vi "ParseCharacters.vi"(11 "TextIn":string) -> (3 "Characters":T1[](array[typedef]))   [LabVIEW 2022 SP3]
uses:
  <vilib>/Utility/error.llb/Trim Whitespace One-Sided.vi
  TypeDefs/Character.ctl
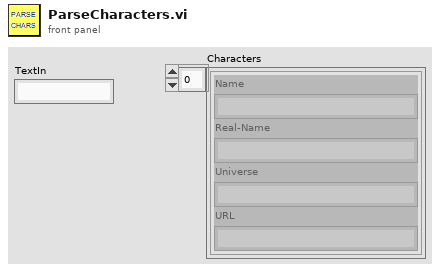
[diagram p1: front panel]
types:
  T1 = typedef "Character.ctl" = cluster{"Name":string, "Real-Name":string, "Universe":string, "URL":string}
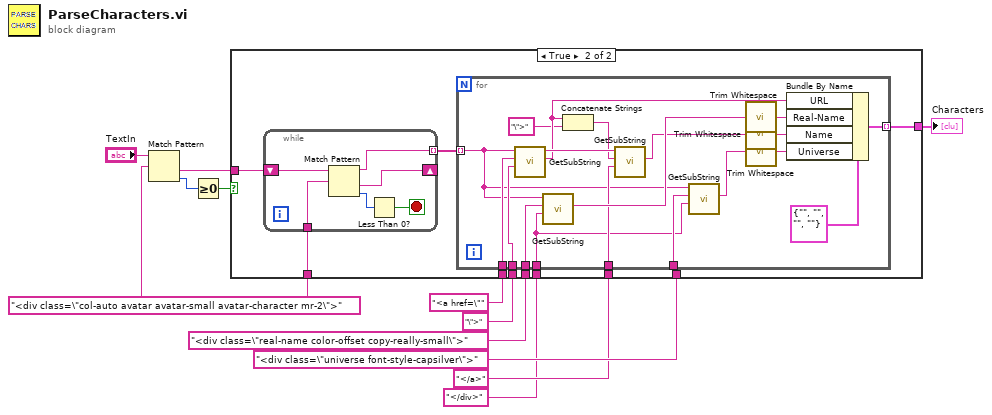
[diagram p0: block diagram]
diagram:
  w3 = "<div class=\"col-auto avatar avatar-small avatar-character mr-2\">" ("End Search")
  n1 = Match Pattern(string="TextIn", regular expression=w3) -> (after substring=w6:string, offset past match=w4:i32)  [unwired: 1 in, 2 out]
  n2 = Greater Or Equal To 0?(x=w4) -> (x >= 0?=w5:bool)
  n3 = case shown="True" w5 {
    tunnel: w3 -> [_ w22]
    tunnel: w6 -> [_ w21]
    tunnel: "<a href=\"" ("End Search") -> [_ w19]
    tunnel: "\">" ("End Search") -> [_ w18]
    tunnel: "<div class=\"real-name color-offset copy-really-small\">" ("End Search") -> [_ w17]
    tunnel: "</div>" ("End Search") -> [_ w16]
    tunnel: "</a>" ("End Search") -> [_ w15]
    tunnel: "<div class=\"universe font-style-capsilver\">" ("End Search") -> [_ w14]
    tunnel: [_ w13] -> w1
    frame False {
    }
    frame True {
      n4 = while {
        shift-right: [w44] -> _
        shift-left: w21 -> [w47]
        tunnel: w22 -> [w46]
        tunnel: [w45] -> w20 mode=indexing
        stop <- w42 stop-if-true
        n5 = Match Pattern(string=w47, regular expression=w46) -> (before substring=w45:string, after substring=w44:string, offset past match=w43:i32)  [unwired: 1 in, 1 out]
        n6 = Less Than 0?(x=w43) -> (x < 0?=w42:bool)
      }
      n7 = for {
        tunnel: w20 -> [w30] mode=indexing
        tunnel: w19 -> [w41]
        tunnel: w18 -> [w40]
        tunnel: w17 -> [w38]
        tunnel: w16 -> [w28]
        tunnel: w15 -> [w32]
        tunnel: w14 -> [w29]
        tunnel: [w26] -> w13 mode=indexing
        n8 = call "GetSubString.vi"("End Search"=w40, "Start Search"=w41, "String In"=w30) -> ("Match"=w35:string, "Following String Out"=w36:string)  [unwired: 6 in, 1 out]
        n9 = call "GetSubString.vi"("End Search"=w28, "Start Search"=w38, "String In"=w30) -> ("Match"=w37:string)  [unwired: 6 in, 2 out]
        n10 = Concatenate Strings(w35, "\">" ("string")) -> (w33:string)
        n11 = call "GetSubString.vi"("End Search"=w32, "Start Search"=w33, "String In"=w36) -> ("Match"=w31:string)  [unwired: 6 in, 2 out]
        n12 = call "GetSubString.vi"("End Search"=w28, "Start Search"=w29, "String In"=w30) -> ("Match"=w27:string)  [unwired: 6 in, 2 out]
        n13 = call <vilib>:"Trim Whitespace.vi"("string"=w37) -> ("trimmed string"=w25:string)  [unwired: 1 in]
        n14 = call <vilib>:"Trim Whitespace.vi"("string"=w31) -> ("trimmed string"=w24:string)  [unwired: 1 in]
        n15 = call <vilib>:"Trim Whitespace.vi"("string"=w27) -> ("trimmed string"=w23:string)  [unwired: 1 in]
        n16 = Bundle By Name(cluster=T1 {"Name"="", "Real-Name"="", "Universe"="", "URL"=""}, "URL"=w35, "Real-Name"=w25, "Name"=w24, "Universe"=w23) -> (w26:T1)
      }
    }
  }
  "Characters" <- w1
